vi "ke37xx TSP Script Loader.vi"(0 "VISA Resource Name":refnum<visa-resource-name>, 5 "TSP Script Name":string, 7 "TSP Script":string, 9 "Run TSP Script (False)":bool, 11 "error in (no error)":errorcluster) -> (4 "VISA Resource Name Out":refnum<visa-resource-name>, 15 "error out":errorcluster)   [LabVIEW 2009, in "Keithley 3700 Series.lvlib"]
doc: "This VI provides a method to download, and optionally run a TSP script on the instrument."
uses:
  <instrlib>/Keithley 3706/Keithley 3700 Series.lvlib
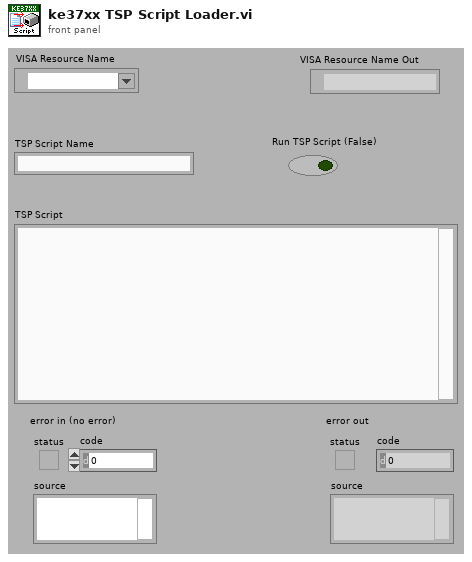
[diagram p1: front panel]
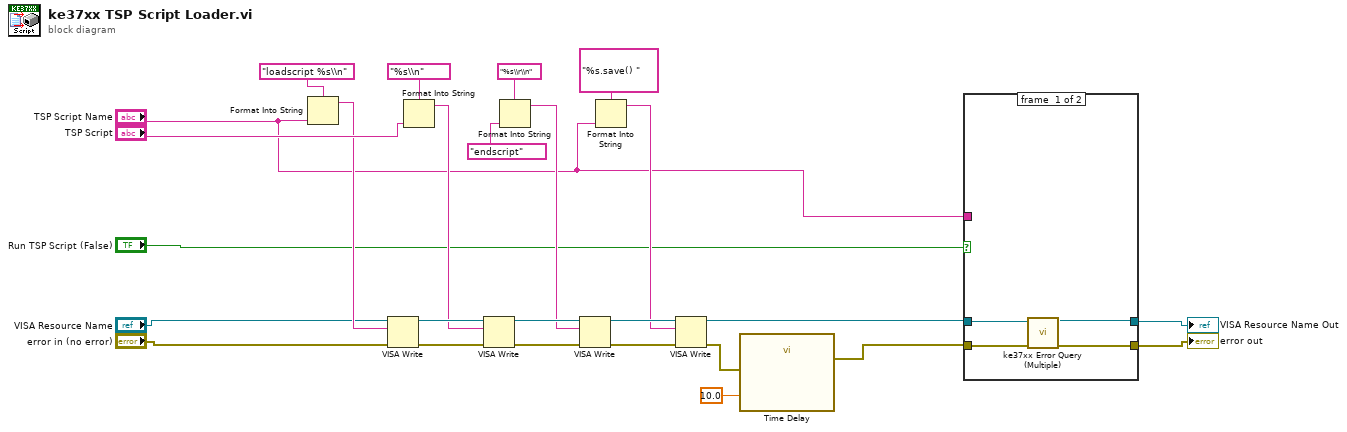
[diagram p0: block diagram]
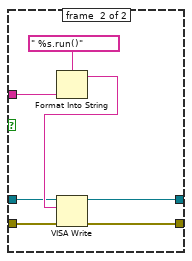
[diagram p2: hidden frame]
diagram:
  n1 = Format Into String(format string="loadscript %s\\n", "TSP Script Name") -> (resulting string=w12:string)  [unwired: 2 in, 1 out]
  n2 = VISA Write(VISA resource name="VISA Resource Name", write buffer=w12, error in (no error)="error in (no error)") -> (VISA resource name out=w20:refnum<visa-resource-name>, error out=w19:errorcluster)  [unwired: 1 out]
  n3 = Format Into String(format string="%s\\n", "TSP Script") -> (resulting string=w11:string)  [unwired: 2 in, 1 out]
  n4 = VISA Write(VISA resource name=w20, write buffer=w11, error in (no error)=w19) -> (VISA resource name out=w18:refnum<visa-resource-name>, error out=w17:errorcluster)  [unwired: 1 out]
  n5 = Format Into String(format string="%s\\r\\n", "endscript") -> (resulting string=w10:string)  [unwired: 2 in, 1 out]
  n6 = VISA Write(VISA resource name=w18, write buffer=w10, error in (no error)=w17) -> (VISA resource name out=w16:refnum<visa-resource-name>, error out=w15:errorcluster)  [unwired: 1 out]
  n7 = Format Into String(format string="%s.save() ", "TSP Script Name") -> (resulting string=w9:string)  [unwired: 2 in, 1 out]
  n8 = VISA Write(VISA resource name=w16, write buffer=w9, error in (no error)=w15) -> (VISA resource name out=w6:refnum<visa-resource-name>, error out=w14:errorcluster)  [unwired: 1 out]
  n9 = call "Time Delay"("error in (no error)"=w14, "Delay Time (s)"=10.0) -> ("error out"=w5:errorcluster)  [unwired: 9 in]
  n10 = case shown="False" "Run TSP Script (False)" {
    tunnel: "TSP Script Name" -> [_ w31]
    tunnel: w6 -> [w30 w35]
    tunnel: w5 -> [w29 w34]
    tunnel: [w27 w32] -> w3
    tunnel: [w28 w33] -> w4
    frame #0 {
      n11 = call <instrlib>:"ke37xx Error Query (Multiple).vi"("VISA resource name"=w30, "error in (no error)"=w29) -> ("VISA resource name out"=w28:refnum<visa-resource-name>, "error out"=w27:errorcluster)  [unwired: 12 out]
    }
    frame #1 {
      n12 = Format Into String(format string=" %s.run()", w31) -> (resulting string=w36:string)  [unwired: 2 in, 1 out]
      n13 = VISA Write(VISA resource name=w35, write buffer=w36, error in (no error)=w34) -> (VISA resource name out=w33:refnum<visa-resource-name>, error out=w32:errorcluster)  [unwired: 1 out]
    }
  }
  "VISA Resource Name Out" <- w4
  "error out" <- w3
